vi "write keys per section.vi"(8 "error in (no error)":errorcluster, 10 "section data":T1, 11 "Refnum in":T2) -> (0 "error out":errorcluster, 3 "Refnum out":T2)   [LabVIEW 2024, in "API Config Files Management.lvlib"]
doc: "This function writes all keys and their corresponding values to a configuration .ini file, given the section name. The input is a cluster containing three elements: a string for the section name, a 1-D string array for the keys, and a 1-D string array for the corresponding values."
uses:
  API Config Files Management.lvlib
  <vilib>/Utility/config.llb/Config Data RefNum.ctl
  section data.ctl
  <vilib>/Utility/config.llb/Write Key (String).vi
  <vilib>/Utility/config.llb/NI_LVConfig.lvlib
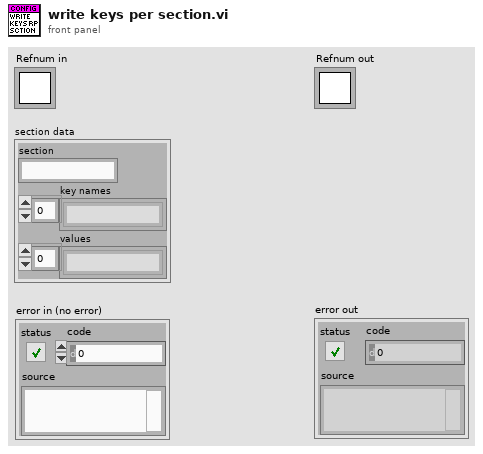
[diagram p1: front panel]
types:
  T1 = typedef "API Config Files Management.lvlib/section data.ctl" = cluster{"section":string, "key names":string[], "values":string[]}
  T2 = typedef "NI_LVConfig.lvlib/Config Data RefNum.ctl" = refnum<k1>
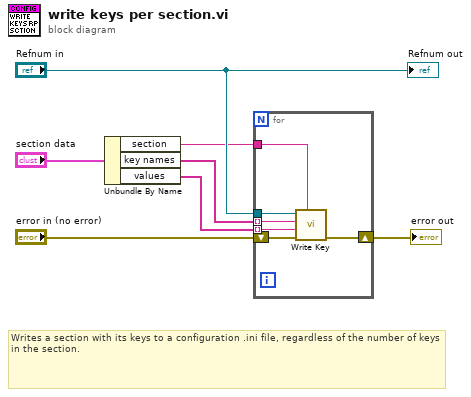
[diagram p0: block diagram]
diagram:
  # "Writes a section with its keys to a configuration .ini file, regardless of the number of keys in the section."
  n1 = Unbundle By Name("section data") -> ("section"=w3:string, "key names"=w2:string[], "values"=w1:string[])
  n2 = for {
    tunnel: "Refnum in" -> [w12]
    tunnel: w3 -> [w11]
    shift-right: [w10] -> w6
    shift-left: "error in (no error)" -> [w13]
    tunnel: w1 -> [w9] mode=indexing
    tunnel: w2 -> [w8] mode=indexing
    n3 = call-poly <vilib>:"Write Key.vi"("section"=w11, "error in (no error)"=w13, "value"=w9, "key"=w8, "refnum"=w12) -> ("error out"=w10:errorcluster)  [unwired: 4 in, 2 out]
  }
  "error out" <- w6
  "Refnum out" <- "Refnum in"
